vi "LSX Get EEP Rom Value.vi"(8 "error in (no error)":errorcluster, 9 "pValue":string, 10 "Offset":u8, 11 "lLSID":i32) -> (0 "error out":errorcluster, 1 "pValue out":string, 3 "function return":i32)   [LabVIEW 2018, in "Tango.lvlib"]
doc: "TANGOAPI int TANGOCALL LSX_GetEEPRomValue (int lLSID, byte Offset, byte *pValue);"
uses:
  Tango.lvlib
  SubVIs/Tango_DLL.dll
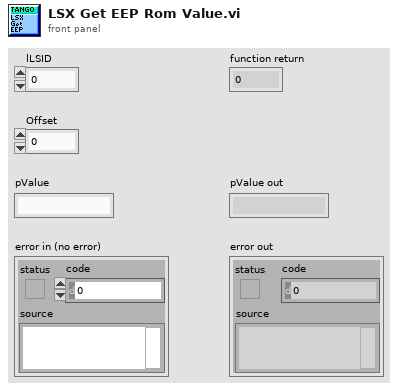
[diagram p1: front panel]
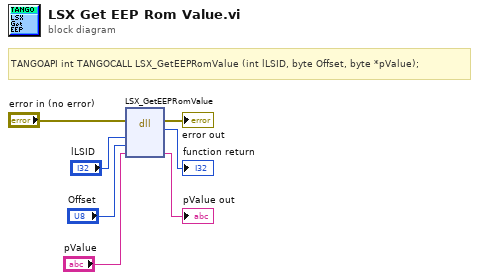
[diagram p0: block diagram]
diagram:
  # "TANGOAPI int TANGOCALL LSX_GetEEPRomValue (int lLSID, byte Offset, byte *pValue);"
  n1 = dll-call lib="C:/Users/Familie/Documents/LabviewIX81/lib/TANGO Stage/SubVIs/Tango_DLL.*" fn="LSX_GetEEPRomValue"(error in="error in (no error)", "lLSID"="lLSID", "Offset"="Offset", "pValue"="pValue") -> (error out=→"error out":errorcluster, →"function return":i32, "pValue"=→"pValue out":string)  [unwired: 4 in, 1 out]
